vi "Update Ctrls Refs.vi"(8 "error in":errorcluster, 10 "Ctrl Sequences":string[](array[string]), 11 "Controls[] in":refnum<vi>[](array[refnum])) -> (0 "error out":errorcluster, 3 "Controls[] out":refnum<vi>[](array[refnum]))   [LabVIEW 2018, in "NISAST VI Scripting.lvlib" / "VI.lvlib" / "Connector.lvlib"]
uses:
  Connector/Connector.lvlib
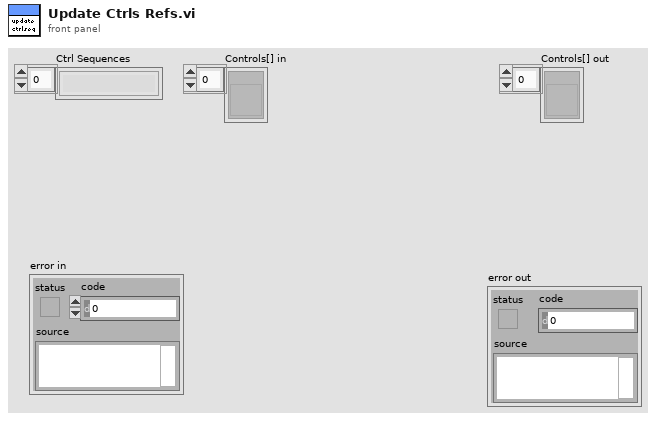
[diagram p1: front panel]
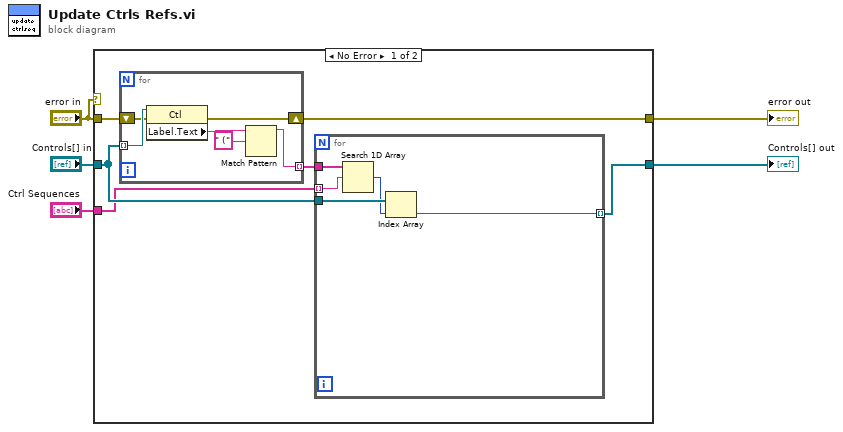
[diagram p0: block diagram]
diagram:
  n1 = case shown="No Error" "error in" {
    tunnel: [w11 w23] -> w5
    tunnel: [w10 w24] -> w4
    tunnel: "error in" -> [w9 w23]
    tunnel: "Controls[] in" -> [w8 w24]
    tunnel: "Ctrl Sequences" -> [w6 _]
    frame No Error {
      n2 = for {
        tunnel: w8 -> [w22] mode=indexing
        tunnel: [w18] -> w7 mode=indexing
        shift-right: [w20] -> w11
        shift-left: w9 -> [w21]
        n3 = property class="Ctl"(reference=w22, error in=w21) -> (error out=w20:errorcluster, "Label.Text"=w19:string)  [unwired: 1 out]
        n4 = Match Pattern(string=w19, regular expression=" (") -> (before substring=w18:string)  [unwired: 4 out]
      }
      n5 = for {
        tunnel: w6 -> [w15] mode=indexing
        tunnel: w7 -> [w16]
        tunnel: w8 -> [w14]
        tunnel: [w12] -> w10 mode=indexing
        n6 = Search 1D Array(1D array=w16, element=w15) -> (index of element=w13:i32)  [unwired: 1 out]
        n7 = Index Array(array=w14, index=w13) -> (element=w12:refnum<vi>)
      }
    }
    frame Error {
    }
  }
  "error out" <- w5
  "Controls[] out" <- w4
